vi "Main.vi"() -> ()   [LabVIEW 2014]
panel:
  in  "element":dbl
  out "error out":errorcluster
  out "failure setting of phases":i32[](array[numeric])
  in  "error in (no error)":errorcluster
  in  "timeout ms (60000)":i32=6000
  in  "remote port or service name":u16=55555
  in  "address":string="10.20.126.62"
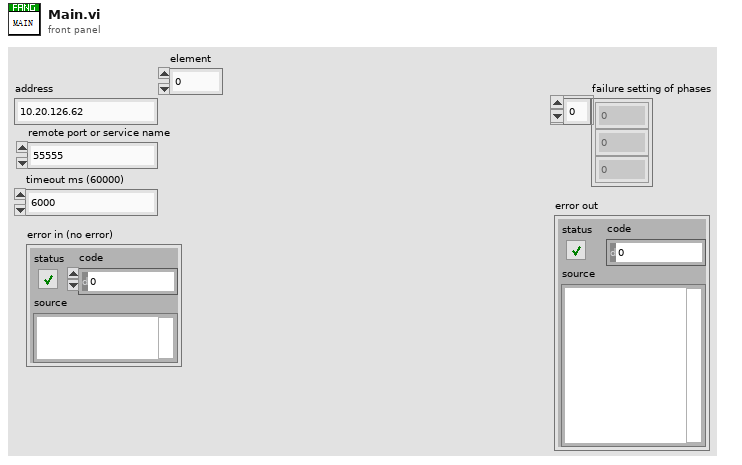
[diagram p1: front panel]
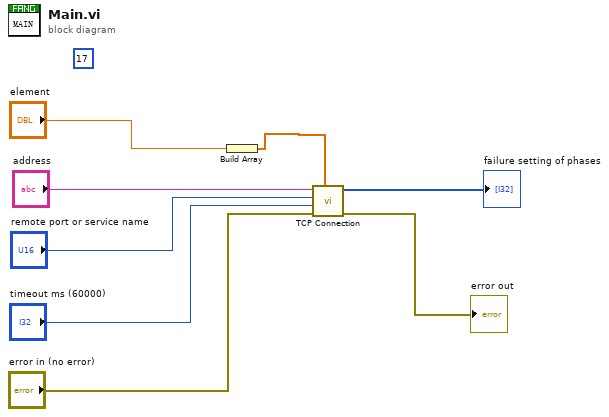
[diagram p0: block diagram]
diagram:
  (unwired) 17
  n1 = Build Array("element") -> (w2:dbl[])
  n2 = call "TCP Connection.vi"("phase shift array"=w2, "error in (no error)"="error in (no error)", "timeout ms (60000)"="timeout ms (60000)", "remote port or service name"="remote port or service name", "address"="address") -> ("error out"=→"error out":errorcluster, "failure setting of phases"=→"failure setting of phases":i32[])  [unwired: 5 in]
